vi "FGV Tester.vi"() -> ()   [LabVIEW 2021]
uses:
  support/Controls/Auto Stats.ctl
  RT/Controls/Auto Times.ctl
  Controls/AVL Auto Time.ctl
  Controls/Logging FGV.ctl
panel:
  in  "Auto Stats":T1
  in  "Enum":enum16{"Start", "Exit Auto", "Update Log"}(ring)=enum."Update Log"
  in  "Continue":bool
  in  "Stop Loop":bool
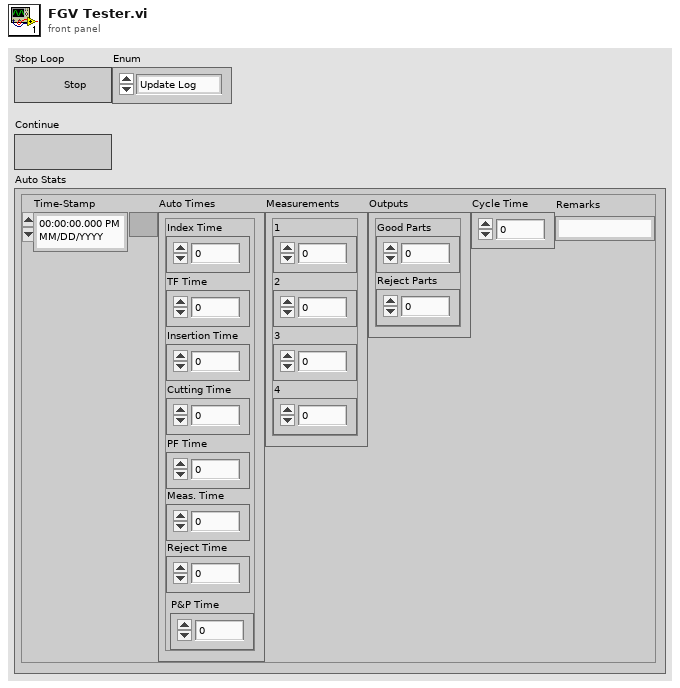
[diagram p1: front panel]
types:
  T1 = typedef "Auto Stats.ctl" = cluster{"Time-Stamp":timestamp, "Auto Times":T2, "Measurements":cluster{"1":dbl, "2":dbl, "3":dbl, "4":dbl}, "Outputs":cluster{"Good Parts":u32, "Reject Parts":u32}, "Cycle Time":dbl, "Remarks":string}
  T2 = typedef "Auto Times.ctl" = cluster{"Index Time":u32, "TF Time":u32, "Insertion Time":u32, "Cutting Time":u32, "PF Time":u32, "Meas. Time":u32, "Reject Time":u32, "P&P Time":u32}
  T3 = typedef "AVL Auto Time.ctl" = enum16{"Start Session", "Exited Auto", "Resumed Auto", "Read Time", "Reload Values"}
  T4 = typedef "Logging FGV.ctl" = enum16{"Start Shift", "Reload Values", "Log Index", "Read Shift", "Close Shift", "Save Values"}
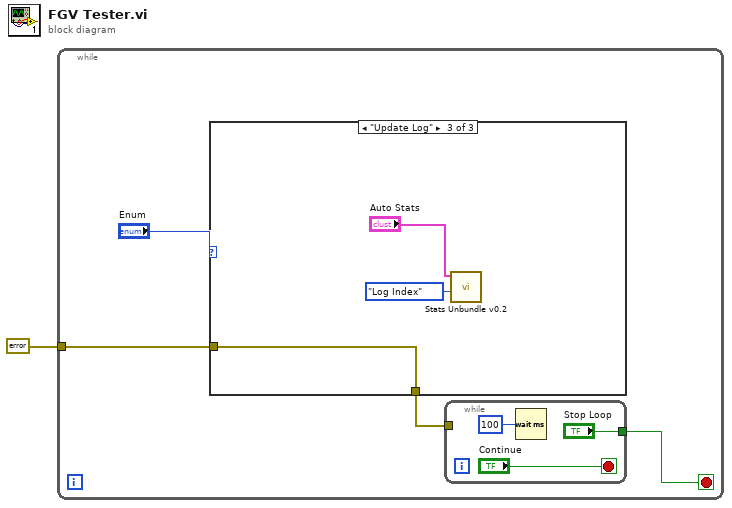
[diagram p0: block diagram]
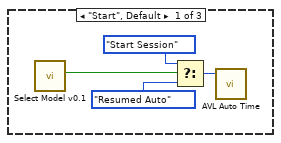
[diagram p2: hidden frame]
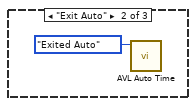
[diagram p3: hidden frame]
diagram:
  n1 = while {
    tunnel: errorcluster {"status"=FALSE, "code"=0, "source"=""} ("error constant") -> [w3]
    stop <- w4 stop-if-true
    n2 = case shown="\"Update Log\"" "Enum" {
      tunnel: w3 -> [_ _ w14]
      tunnel: [_ _ w14] -> w2
      frame "Start", Default {
        n3 = call "Select Model v0.1.vi"() -> ("Refresh Indicators?"=w12:bool)  [unwired: 9 in, 2 out]
        n4 = Select(t=AVL_Auto_Time."Start Session" ("State"), s=w12, f=AVL_Auto_Time."Resumed Auto" ("State")) -> (s? t:f=w9:T3)
        n5 = call "AVL Auto Time.vi"("State"=w9) -> ()  [unwired: 10 in, 1 out]
      }
      frame "Exit Auto" {
        n6 = call "AVL Auto Time.vi"("State"=AVL_Auto_Time."Exited Auto") -> ()  [unwired: 10 in, 1 out]
      }
      frame "Update Log" {
        n7 = call "Stats Unbundle v0.2.vi"("State"=Logging_FGV."Log Index", "Auto Stats"="Auto Stats") -> ()  [unwired: 3 in, 7 out]
      }
    }
    n8 = while {
      tunnel: ["Stop Loop"] -> w4
      tunnel: w2 -> [_]
      stop <- "Continue" stop-if-true
      n9 = Wait (ms)(milliseconds to wait=u32 100) -> ()  [unwired: 1 out]
    }
  }
